vi "Load_and_play_audio signal.vi"() -> ()   [LabVIEW 2024]
uses:
  <vilib>/sound2/lvsound2.llb/Sound Data Format.ctl
  <vilib>/sound2/lvsound2.llb/Sampling Mode.ctl
  <vilib>/sound2/lvsound2.llb/Sound File Read Open.vi
  <vilib>/sound2/lvsound2.llb/Sound File Info (refnum).vi
  <vilib>/sound2/lvsound2.llb/Sound File Read (DBL).vi
  <vilib>/sound2/lvsound2.llb/Sound Output Write (DBL).vi
panel:
  in  "path":path
  out "Waveform Graph 2":waveform(dbl)[](graph)
  in  "?":bool
  in  "number of samples/ch":i32=10000
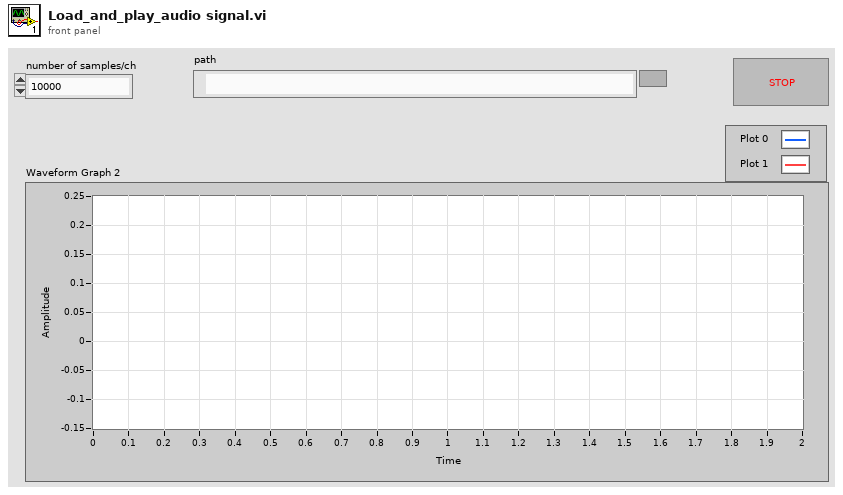
[diagram p1: front panel]
types:
  T1 = typedef "Sampling Mode.ctl" = i32
  T2 = typedef "Sound Data Format.ctl" = cluster{"sample rate (S/s)":dbl, "number of channels":i32, "bits per sample":i32}
  T3 = typedef "Sound File Refnum.ctl" = refnum<file>
  T4 = typedef "Sound Output Task ID.ctl" = u32
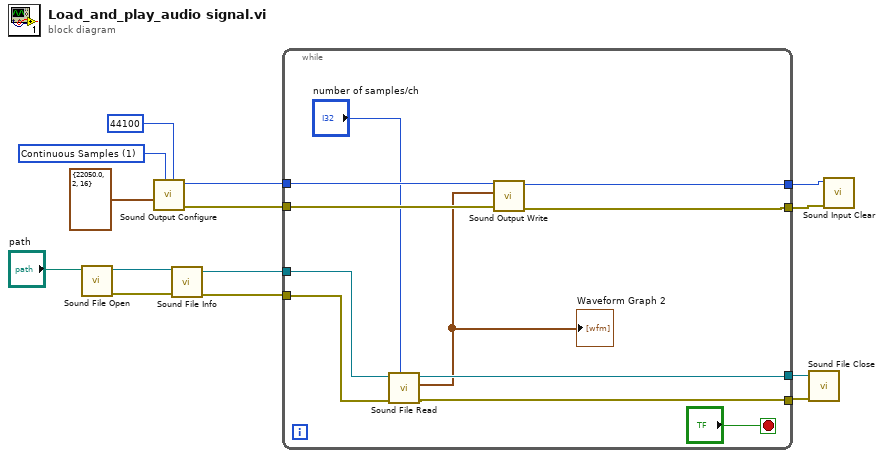
[diagram p0: block diagram]
diagram:
  w14 = T1 1 items=["Finite Samples", "Continuous Samples"] ("sample mode")
  n1 = call-poly <vilib>:"Sound File Open.vi"("path"="path") -> ("error out"=w3:errorcluster, "sound file refnum"=w4:T3)  [unwired: 9 in]
  n2 = call <vilib>:"Sound Output Configure.vi"("number of samples/ch"=44100, "sample mode"=w14, "sound format"=T2 {"sample rate (S/s)"=22050.0, "number of channels"=2, "bits per sample"=16}) -> ("error out"=w12:errorcluster, "task ID"=w11:T4)  [unwired: 7 in]
  n3 = call-poly <vilib>:"Sound File Info.vi"("error in (no error)"=w3, "sound file refnum"=w4) -> ("error out"=w2:errorcluster, "sound file refnum out"=w1:T3)  [unwired: 6 in, 2 out]
  n4 = while {
    tunnel: w12 -> [w25]
    tunnel: [w23] -> w9
    tunnel: [w22] -> w10
    tunnel: w11 -> [w21]
    tunnel: w1 -> [w20]
    tunnel: w2 -> [w19]
    tunnel: [w18] -> w7
    tunnel: [w17] -> w6
    stop <- "?" stop-if-true
    n5 = call-poly <vilib>:"Sound File Read.vi"("number of samples/ch (-1: all)"="number of samples/ch", "error in (no error)"=w19, "sound file refnum"=w20) -> ("error out"=w17:errorcluster, "data"=w15:waveform(dbl)[], "sound file refnum out"=w18:T3)  [unwired: 4 in, 2 out]
    "Waveform Graph 2" <- w15
    n6 = call-poly <vilib>:"Sound Output Write.vi"("error in (no error)"=w25, "data"=w15, "task ID"=w21) -> ("error out"=w23:errorcluster, "task ID out"=w22:T4)  [unwired: 7 in]
  }
  n7 = call <vilib>:"Sound File Close.vi"("error in (no error)"=w6, "sound file refnum"=w7) -> ()  [unwired: 9 in, 1 out]
  n8 = call <vilib>:"Sound Input Clear.vi"("error in (no error)"=w9, "task ID"=w10) -> ()  [unwired: 9 in, 1 out]
